vi "Set Button References.vi"(8 "error in":errorcluster, 9 "label array in":string[](array[string]), 10 "controls[] in":refnum<vi>[](array[refnum]), 11 "UI Data in":T1={"SR Display List"=[], "Filter Cluster"={"Show Resolved"=TRUE, "Show Potentially Resolved"=TRUE, "Show Passoffs"=TRUE, "Show In Collab"=TRUE}, "Exit"=refnum, "Main VI"=refnum, "Sorting"=enum."SR Status", "Message"=refnum, "Legend"=refnum, "Sorting Reference"=refnum, "SR Display List Reference"=refnum, "Filter Cluster Reference"=refnum, "Remove SR"=refnum, "Add SR"=refnum, "Refresh SRs"=refnum} {"SR Display List"."Creation Date" format="%<%x>T"; "SR Display List"."Last Updated" format="%<%x>T"}) -> (0 "error out":errorcluster, 3 "UI Data out":T1={"SR Display List"=[], "Filter Cluster"={"Show Resolved"=TRUE, "Show Potentially Resolved"=TRUE, "Show Passoffs"=TRUE, "Show In Collab"=TRUE}, "Exit"=refnum, "Main VI"=refnum, "Sorting"=enum."SR Status", "Message"=refnum, "Legend"=refnum, "Sorting Reference"=refnum, "SR Display List Reference"=refnum, "Filter Cluster Reference"=refnum, "Remove SR"=refnum, "Add SR"=refnum, "Refresh SRs"=refnum} {"SR Display List"."Creation Date" format="%<%x>T"; "SR Display List"."Last Updated" format="%<%x>T"})   [LabVIEW 2018]
uses:
  Type Defs/UI Loop Data.ctl
  Type Defs/SR Cluster.ctl
  Type Defs/SR Status.ctl
  Type Defs/Filter Cluster.ctl
  Type Defs/Sorting Methods.ctl
  Type Defs/SR Display List Reference.ctl
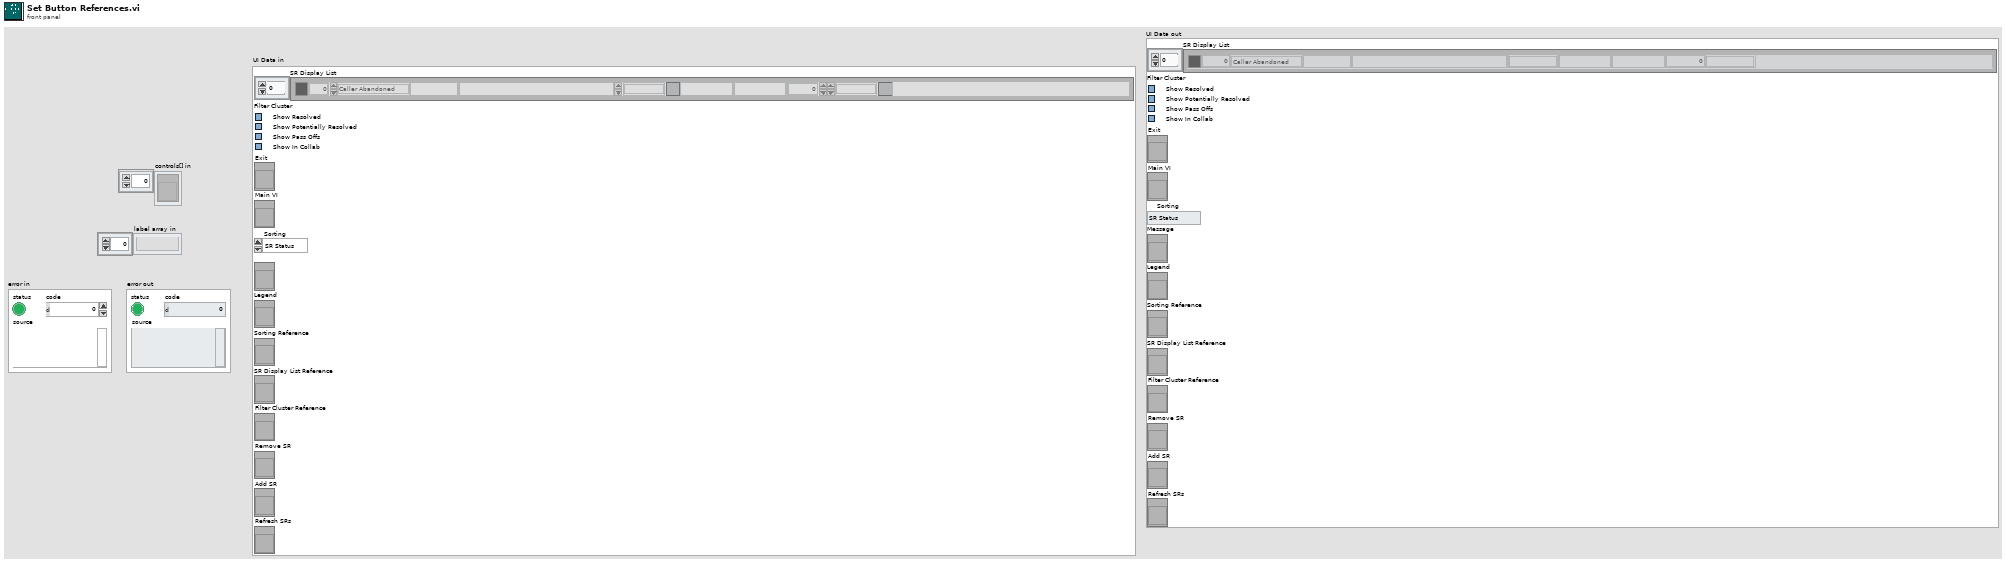
[diagram p1: front panel]
types:
  T1 = typedef "UI Loop Data.ctl" = cluster{"SR Display List":T2[], "Filter Cluster":T4, "Exit":refnum<vi>, "Main VI":refnum<vi>, "Sorting":T5, "Message":refnum<vi>, "Legend":refnum<vi>, "Sorting Reference":refnum<vi>, "SR Display List Reference":T6, "Filter Cluster Reference":refnum<vi>, "Remove SR":refnum<vi>, "Add SR":refnum<vi>, "Refresh SRs":refnum<vi>}
  T2 = typedef "SR Cluster.ctl" = cluster{"Color":u32, "SR Number":i32, "SR Status":T3, "Name":string, "Summary":string, "Last Updated":timestamp, "SR Type":string, "Service Level":string, "Days Open":dbl, "Creation Date":timestamp, "Owner":string, "Note":string}
  T3 = typedef "SR Status.ctl" = enum16{"Caller Abandoned", "Created in Error", "Expired", "Forum Resolved AE", "Forum Resolved Customer", "IN WORK", "IN WORK Collab with AES", "IN WORK Collab with PSE", "IN WORK Collab with SE", "IN WORK Customer Added Note", "IN WORK Escalation", "IN WORK Wait on Customer", "Open", "Potentially Resolved", "Presumed Resolved", "RMA Approved for Return", "RMA Closed", "RMA Closed - DOA", "RMA In Progress", "RMA Open", "RMA Waiting on Customer", "Resolved", "Passed Off"}
  T4 = typedef "Filter Cluster.ctl" = cluster{"Show Resolved":bool, "Show Potentially Resolved":bool, "Show Passoffs":bool, "Show In Collab":bool}
  T5 = typedef "Sorting Methods.ctl" = enum16{"SR Status", "Most Recent", "SR Type", "SR Number", "Days Open", "Urgency"}
  T6 = typedef "SR Display List Reference.ctl" = refnum<vi>
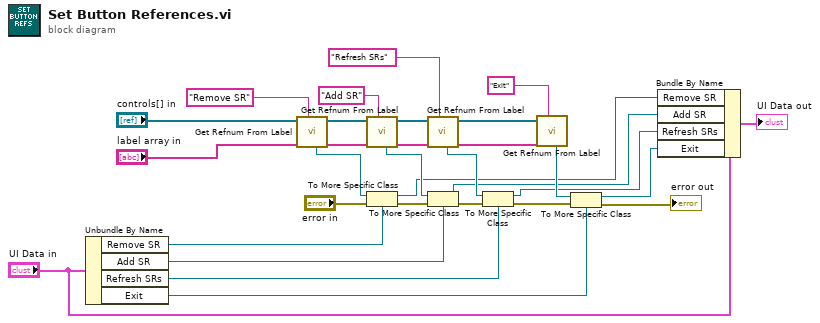
[diagram p0: block diagram]
diagram:
  n1 = Unbundle By Name("UI Data in") -> ("Remove SR"=w10:refnum<vi>, "Add SR"=w9:refnum<vi>, "Refresh SRs"=w8:refnum<vi>, "Exit"=w7:refnum<vi>)
  n2 = call "Get Refnum From Label.vi"("label"="Remove SR", "label array in"="label array in", "controls[] in"="controls[] in") -> ("label array out"=w23:string[], "controls[] out"=w18:refnum<vi>[], "refnum out"=w28:refnum<vi>)  [unwired: 6 in]
  n3 = call "Get Refnum From Label.vi"("label"="Add SR", "label array in"=w23, "controls[] in"=w18) -> ("label array out"=w22:string[], "controls[] out"=w17:refnum<vi>[], "refnum out"=w27:refnum<vi>)  [unwired: 6 in]
  n4 = To More Specific Class(target class=w10, reference=w28, error in="error in") -> (specific class reference=w2:refnum<vi>, error out=w20:errorcluster)
  n5 = call "Get Refnum From Label.vi"("label"="Refresh SRs", "label array in"=w22, "controls[] in"=w17) -> ("label array out"=w14:string[], "controls[] out"=w16:refnum<vi>[], "refnum out"=w26:refnum<vi>)  [unwired: 6 in]
  n6 = To More Specific Class(target class=w9, reference=w27, error in=w20) -> (specific class reference=w3:refnum<vi>, error out=w21:errorcluster)
  n7 = To More Specific Class(target class=w8, reference=w26, error in=w21) -> (specific class reference=w4:refnum<vi>, error out=w12:errorcluster)
  n8 = call "Get Refnum From Label.vi"("label"="Exit", "label array in"=w14, "controls[] in"=w16) -> ("refnum out"=w13:refnum<vi>)  [unwired: 6 in, 2 out]
  n9 = To More Specific Class(target class=w7, reference=w13, error in=w12) -> (specific class reference=w5:refnum<vi>, error out=→"error out":errorcluster)
  n10 = Bundle By Name(cluster="UI Data in", "Remove SR"=w2, "Add SR"=w3, "Refresh SRs"=w4, "Exit"=w5) -> (→"UI Data out":T1)
